vi "Dashboard Main.vi"() -> ()   [LabVIEW 2017]
uses:
  <vilib>/Utility/miscctls.llb/LVRowAndColumnTypeDef.ctl
  <vilib>/event_ctls.llb/eventvkey.ctl
  <vilib>/Rock Robotics/Network Tables/NT Read Numeric Array.vi
  <vilib>/Rock Robotics/WPI/Dashboard/WPI_DashboardLogging Global.vi
panel:
  in  "Camera Settings Right":T1={"Frame Rate"=30, "Compression"=30, "Size"=1, "DB Camera Config"=FALSE} {"Frame Rate" scale=1.0..30.0; "Compression" scale=100.0..-1.0; "Size" items=["640x480", "320x240", "160x120"]}
  in  "Camera Name Right":string(combo)="No Camera Selection"
  out "Camera Info":cluster{"Mbps LED":bool, "Mbps":dbl, "fps":dbl} {"fps" format="%#.1g"; "Mbps" format="%#.1g"}
  in  "Camera Settings":T1={"Frame Rate"=30, "Compression"=30, "Size"=1, "DB Camera Config"=FALSE} {"Frame Rate" scale=1.0..30.0; "Compression" scale=100.0..-1.0; "Size" items=["640x480", "320x240", "160x120"]}
  in  "TCP":refnum<k5>
  in  "Rec Mode":enum32{"Stop", "Record", "Playback"}(radio)
  out "Robot IP":string
  out "Image Message":string="Timeout in Camera Communications"
  in  "Dashboard Tab":T2(tab)=enum."Custom"
  in  "Select Auto":string(combo)="Select Autonomous ..."
  out "NT Connection":bool
  out "MotorChart R":cluster{"Numeric":dbl, "Numeric":dbl}(graph)
  out "MotorChart L":cluster{"Numeric":dbl, "Numeric":dbl}(graph)
  out "MotorSliders R":cluster{"MotorSlide1":dbl, "MotorSlide2":dbl} {"MotorSlide2" scale=-1.0..1.0 scale format="%#_2e"; "MotorSlide1" scale=-1.0..1.0 scale format="%#_2e"}
  out "MotorSliders L":cluster{"MotorSlide1":dbl, "MotorSlide2":dbl} {"MotorSlide2" scale=-1.0..1.0 scale format="%#_2e"; "MotorSlide1" scale=-1.0..1.0 scale format="%#_2e"}
  out "Gyro":dbl(knob) scale=0.0..360.0
  out "JS1 Z":dbl(slide) scale=-1.0..1.0 scale format="%#_2e"
  out "JS1 Graph":cluster{"X":dbl, "Y":dbl}[](graph)
  out "JS1 Buttons":T3
  out "JS2 Z":dbl(slide) scale=-1.0..1.0 scale format="%#_2e"
  out "JS2 Graph":cluster{"X":dbl, "Y":dbl}[](graph)
  out "JS2 Buttons":T3
  out "Mode":T4(ring)=enum."Auto Disabled"
  out "Camera Image Right":T5(plugin-control)
  in  "DB/String 9":string
  in  "DB/String 8":string
  in  "DB/String 7":string
  in  "DB/String 6":string
  in  "DB/String 5":string
  in  "DB/String 4":string
  in  "DB/String 3":string
  in  "DB/String 2":string
  in  "DB/String 1":string
  in  "DB/String 0":string
  in  "DB/Slider 0":dbl(slide) scale=0.0..5.0
  in  "DB/Slider 1":dbl(slide) scale=0.0..5.0
  in  "DB/Slider 2":dbl(slide) scale=0.0..5.0
  in  "DB/Slider 3":dbl(slide) scale=0.0..5.0
  out "DB/LED 3":bool
  out "DB/LED 2":bool
  out "DB/LED 1":bool
  out "DB/LED 0":bool
  in  "DB/Button 3":bool
  in  "DB/Button 2":bool
  in  "DB/Button 1":bool
  in  "DB/Button 0":bool caption="New Name"
  in  "Turning Deadband":dbl
  in  "Turning Rate":dbl
  in  "Speed Deadband":dbl
  in  "Speed Rate":dbl
  in  "Climb Time":dbl
  in  "Climb Setpoint":dbl=0.7
  in  "Button Lower Arm Time":dbl
  in  "Button Lower Arm Setpoint":dbl=0.7
  in  "Button Lift Arm Time":dbl
  in  "Button Lift Arm Setpoint":dbl=0.7
  in  "Release Time":dbl
  in  "Release Setpoint":dbl=0.7
  in  "Grab Setpoint":dbl=0.7
  in  "Grab Time":dbl=1.0
  in  "Test Slider":dbl(slide) scale=0.0..100.0 scale format="%#_3g"
  in  "On/Off":bool caption="Solenoid"
  in  "Test Name":u16(ring) items=["Select the test to run..."]
  in  "Test Tree":string(tree)
  in  "Motor":cluster{"Value":dbl, "Enable":bool} {"Value" scale=-1.0..1.0 scale format="%#_3g"}
  out "Progress":T6 {"Test Progress" scale=0.0..100.0}
  in  "Rev/Fwd":cluster{"Forward":bool, "Reverse":bool}
  in  "Test Ring":u16(ring) items=["Monochrome", "Color"]
  out "Cmd Status":string
  in  "Execute Command":bool
  in  "Command Params":string[][](table)
  in  "Command Selection":i32(listbox)
  in  "CheckList":i32(listbox)
  out "Tree":string(tree)
  out "Camera Image":T5(plugin-control)
  out "Background":bool
  in  "Camera Name":string(combo)="No Camera Selection"
  # "HW"
  # "HW"
  # "Joysticks"
  # "Drive Motors"
  # "Front"
  # "Right"
  # "Left"
  # "Back"
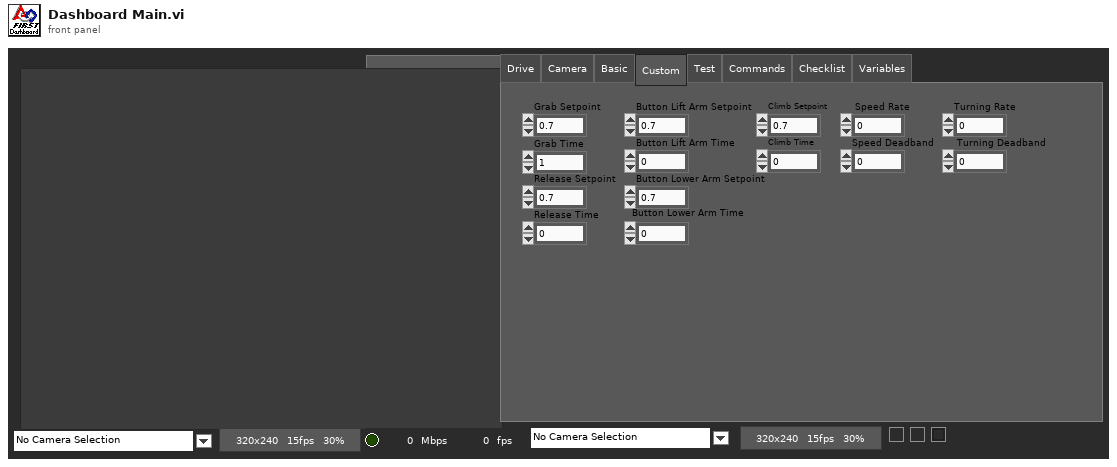
[diagram p1: front panel]
types:
  T1 = cluster{"Frame Rate":i32, "Compression":i32, "Size":u16, "DB Camera Config":bool}
  T2 = enum32{"Drive", "Camera", "Basic", "Custom", "Test", "Commands", "Checklist", "Variables"}
  T3 = cluster{bool, bool, bool, bool, bool, bool, bool, bool, bool, bool, bool, bool}
  T4 = enum8{"Tele-Op Disabled", "Tele-Op Enabled", "Auto Disabled", "Auto Enabled", "Test Disabled", "Test Enabled", "Disconnected", "No Code", "E-Stop"}
  T5 = typedef "IMAQ Image.ctl" = refnum<image>
  T6 = cluster{"Test Progress":u8, "Test Progress Text":string}
  T7 = cluster{"Save Path":path, "Interval (s)":dbl, "Keep":i32}
  T8 = typedef "Image Type" = u32
  T9 = cluster{"IDs":cluster{"RPC field ID":u16, "Unique ID":u16}, "String":string}
  T10 = cluster{"Error Strings":string, "Disable Counts":cluster{u16, u16}, "Rail Faults":cluster{u16, u16, u16}, "Robot IP":string, "DB Mode":u8, "Event Info":cluster{"Name":string, "Type":u8, "Number":u16, "Replay":u8}}
  T11 = cluster{"Storage":cluster{"Disk Free":u64, "RAM Block":u32, "RAM free":u32}, "CPU Utilization":cluster{"CPU % ISR":sgl, "CPU % Time Crit":sgl, "CPU % Timed Str":sgl, "CPU % High":sgl, "CPU % Above":sgl, "CPU % Normal":sgl, "CPU % Low":sgl}, "CAN":cluster{"% Bus Utilization":sgl, "Bus Off Cnt":u32, "TX_FIFO Full Cnt":u32, "Receive Error Cnt":u8, "Transmit Error Cnt":u8}, "HID":cluster{"HID Outputs":u32, "Rumble Low":u16, "Rumble High":u16}[]}
  T12 = cluster{"Status bits":cluster{"Test Mode":bool, "Autonomous":bool, "Enabled":bool, "Code Start":bool, "Brownout":bool, "Reserved 2":bool, "Reserved 3":bool, "E-Stop":bool}, "Code Trace":cluster{"Disabled":bool, "TeleOp":bool, "Auto":bool, "Test":bool}, "Controller Type":enum16{"unknown", "cRIO", "roboRio"}, "Code?":enum16{"unknown", "noCode", "code"}, "Battery V":dbl}
  T13 = cluster{"Control Bits":cluster{"TestMode":bool, "Autonomous":bool, "Enabled":bool, "FMS Present":bool, bool, bool, bool, "E-Stop":bool}, "Team Station ":u8, "Countdown":sgl, "Joystick Values":cluster{"Axes":dbl[], "Buttons":bool[], "POVs":i16[]}[]}
  T14 = cluster{"Axes":dbl[], "Buttons":bool[], "POVs":i16[]}[]
  T15 = cluster{"Axes":dbl[], "Buttons":bool[], "POVs":i16[]}
  T16 = cluster{"Buttons[0]":bool, "Buttons[1]":bool, "Buttons[2]":bool, "Buttons[3]":bool, "Buttons[4]":bool, "Buttons[5]":bool, "Buttons[6]":bool, "Buttons[7]":bool, "Buttons[8]":bool, "Buttons[9]":bool, "Buttons[10]":bool, "Buttons[11]":bool}
  T17 = cluster{"Camera Image":refnum<vi>, "Dashboard Tab":refnum<vi>, "Background":refnum<vi>, "Rec Mode":refnum<vi>, "Test Slider":refnum<vi>, "On/Off ":refnum<vi>, "Test Ring":refnum<vi>, "Rev/Fwd":refnum<vi>, "Test Name":refnum<vi>, "Motor":refnum<vi>, "Progress":refnum<vi>, "CheckList":refnum<vi>, "Tree":refnum<vi>, "Test Tree":refnum<vi>, "Command Params":refnum<vi>, "Command Selection":refnum<vi>, "Execute Command":refnum<vi>, "Cmd Status":refnum<vi>, "Camera Settings":refnum<vi>, "Camera Name":refnum<vi>, "Camera Info":refnum<vi>, "Camera Settings Right":refnum<vi>, "Camera Name Right":refnum<vi>, "Camera Image Right":refnum<vi>}
  T18 = cluster{"Camera Name":string, string, "Saved DB Images Info":cluster{"Save Path":path, "Interval (s)":dbl, "Keep":i32}}
  T19 = cluster{"Camera Name Right":string, string, "Saved DB Images Info":cluster{"Save Path":path, "Interval (s)":dbl, "Keep":i32}}
  T20 = cluster{"Operation":enum16{"Update", "Clear"}, "Color Box":u32}[]
  T21 = typedef "eventvkey.ctl" = enum16{"ASCII", "Enter", "Return", "Shift", "Ctrl", "Alt", "Cmd", "Opt", "Caps", "NumLock", "Clear", "Break", "Up", "Down", "Left", "Right", "Insert", "Delete", "Home", "End", "PageUp", "PageDown", "Escape", "Help", "Pause", "ScrollLock", "F1", "F2", "F3", "F4", "F5", "F6", "F7", "F8", "F9", "F10", "F11", "F12", "F13", "F14", "F15", "F16", "F17", "F18", "F19", "F20", "F21", "F22", "F23", "F24", "Play", "VolumeUp", "VolumeDown", "Mute", "Two Byte Char"}
  T22 = cluster{"Image Size":bool, "Image Type":bool, "Pixel Value":bool, "ROI Information":bool, "Zoom Factor":bool}
  T23 = cluster{"Operation":enum16{"Update", "Clear"}, "Color Box":u32}
  T24 = typedef "LVRowAndColumnTypeDef.ctl" = cluster{"Row":i32, "Column":i32}
  T25 = cluster{"Shift":bool, "Ctrl":bool, "Alt":bool, "Cmd":bool, "Opt":bool}
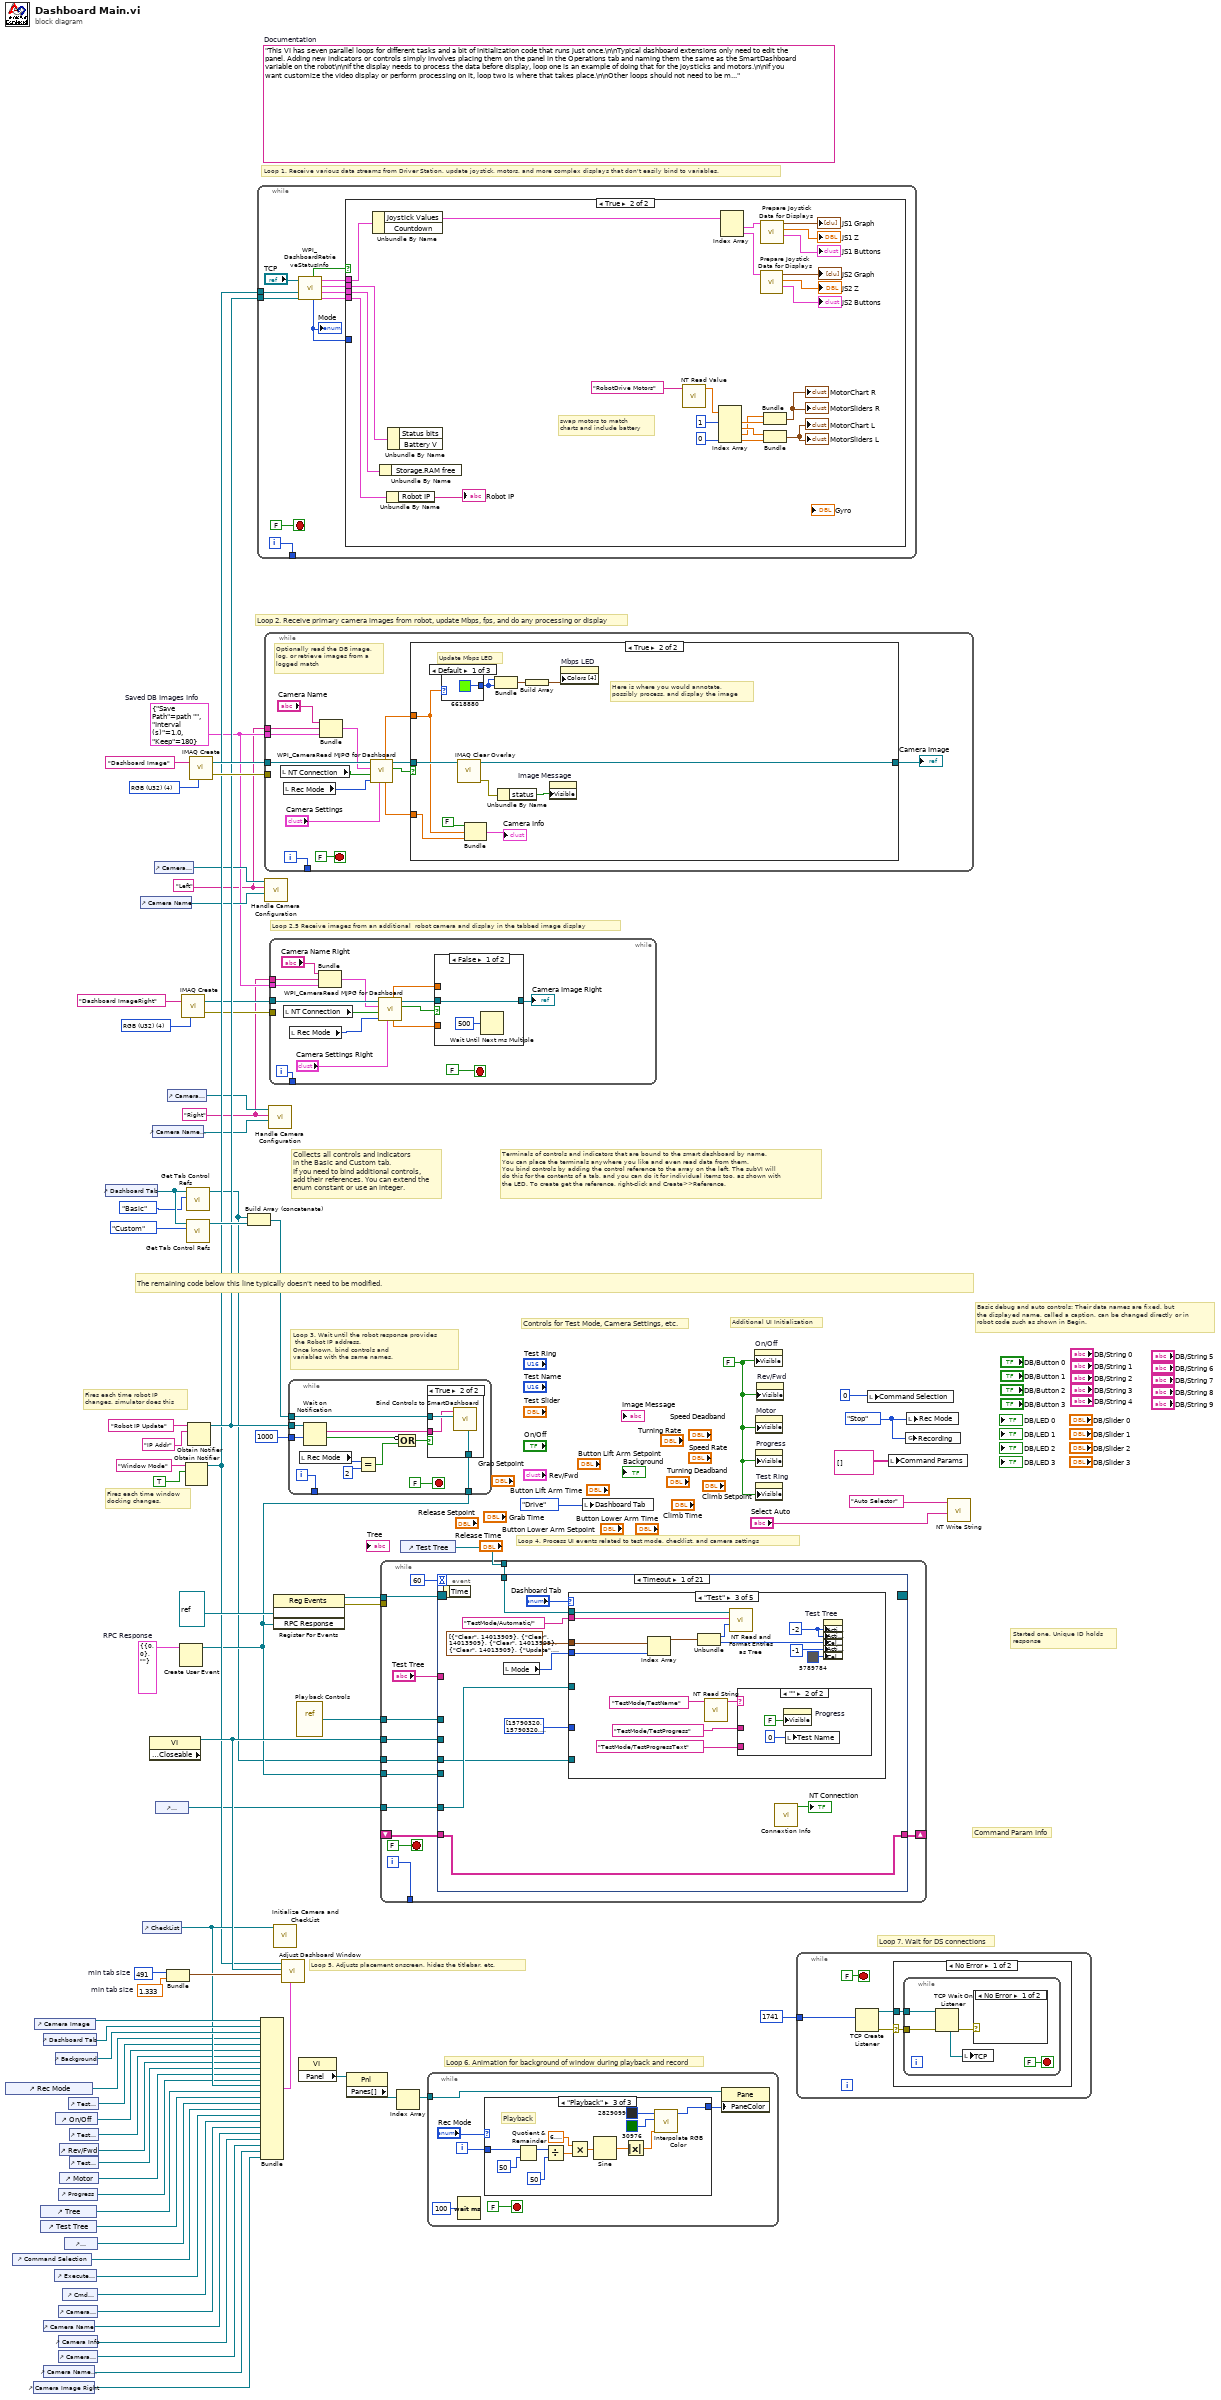
[diagram p0: block diagram]
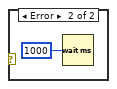
[diagram p3: hidden frame]
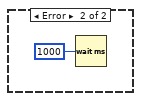
[diagram p4: hidden frame]
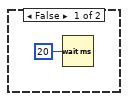
[diagram p5: hidden frame]
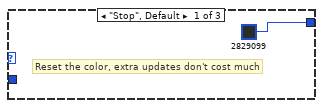
[diagram p6: hidden frame]
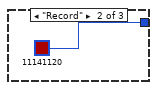
[diagram p7: hidden frame]
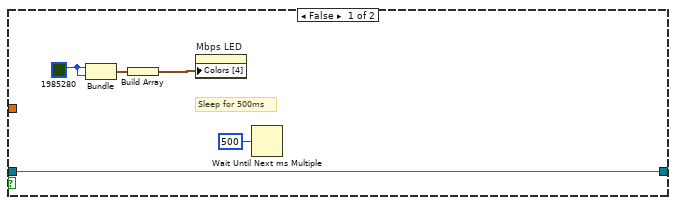
[diagram p9: hidden frame]
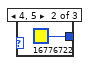
[diagram p10: hidden frame]
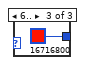
[diagram p11: hidden frame]
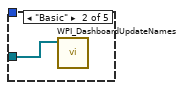
[diagram p13: hidden frame]
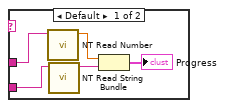
[diagram p14: hidden frame]
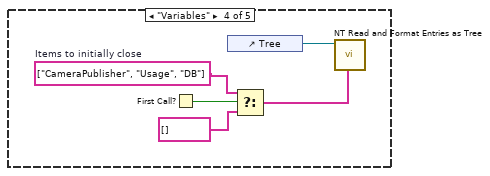
[diagram p15: hidden frame]
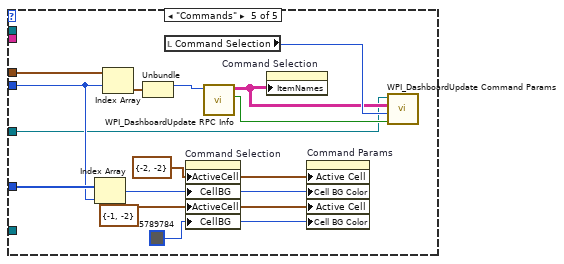
[diagram p16: hidden frame]
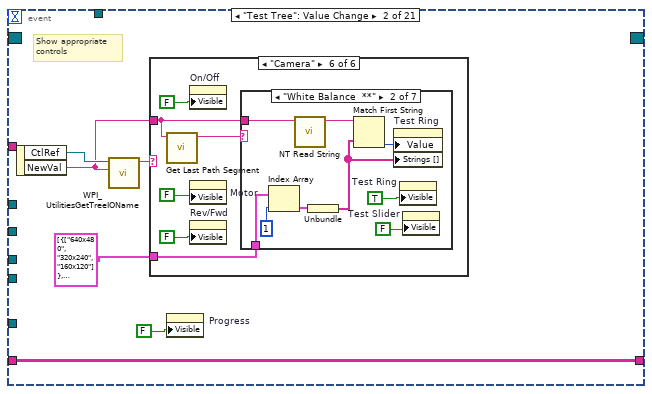
[diagram p17: hidden frame]
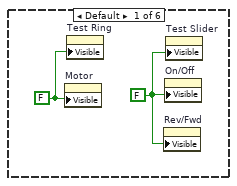
[diagram p18: hidden frame]
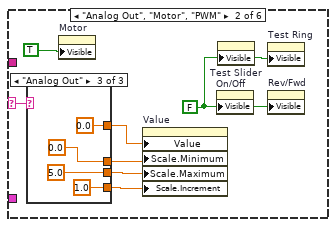
[diagram p19: hidden frame]
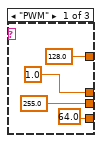
[diagram p20: hidden frame]
diagram:
  w3 = T7 {"Save Path"=path "", "Interval (s)"=1.0, "Keep"=180}  # Saved DB Images Info
  w2 = "Right"
  w1 = "Left"
  w13 = T8 4 items=["Grayscale (U8)", "Grayscale (I16)", "Grayscale (SGL)", "Complex (CSG)", "RGB (U32)", "HSL (U32)", "RGB (U64)"] ("Image Type")
  w29 = T9 {"IDs"={"RPC field ID"=0, "Unique ID"=0}, "String"=""}  # RPC Response
  w52 = 491  # min tab size
  w51 = 1.333  # min tab size
  w59 = enum32{"Stop", "Record", "Playback"}."Stop" ("Rec Mode")
  w36 = FALSE ("Visible")
  (unwired) "This VI has seven parallel loops for different tasks and a bit of initialization code that runs just once.\n\nTypical dashboard extensions only need to edit the panel. Adding new indicators or controls simply involves placing them on the panel in the Operations tab and naming them the same as the SmartDashboard variable on the robot\n\nIf the display needs to process the data before display, loop one is an example of doing that for the joysticks and motors.\n\nIf you want customize the video display or perform processing on it, loop two is where that takes place.\n\nOther loops should not need to be modified. They are pretty standard, and document the task they perform."  # Documentation
  w76 = T8 4 items=["Grayscale (U8)", "Grayscale (I16)", "Grayscale (SGL)", "Complex (CSG)", "RGB (U32)", "HSL (U32)", "RGB (U64)"] ("Image Type")
  # "Loop 2.5 Receive images from an additional  robot camera and display in the tabbed image display"
  # "Command Param Info"
  # "Started one, Unique ID holds\nresponse"
  # "Loop 7. Wait for DS connections"
  # "Basic debug and auto controls: Their data names are fixed, but\nthe displayed name, called a caption, can be changed directly or in\nrobot code such as shown in Begin."
  # "Controls for Test Mode, Camera Settings, etc."
  # "Additional UI Initialization"
  # "Loop 6. Animation for background of window during playback and record"
  # "Fires each time robot IP\nchanges, simulator does this"
  # "Fires each time window\ndocking changes."
  # "Collects all controls and indicators\nin the Basic and Custom tab.\nIf you need to bind additional controls,\nadd their references. You can extend the\nenum constant or use an integer."
  # "The remaining code below this line typically doesn't need to be modified."
  # "Loop 4. Process UI events related to test mode, checklist, and camera settings"
  # "Terminals of controls and indicators that are bound to the smart dashboard by name.\nYou can place the terminals anywhere you like and even read data from them.\nYou bind controls by adding the control reference to the array on the left. The subVI will\ndo this for the contents of a tab, and you can do it for individual items too, as shown with\nthe LED. To create get the reference, right-click and Create>>Reference."
  # "Loop 3. Wait until the robot response provides\n the Robot IP address.\nOnce known, bind controls and\nvariables with the same names."
  # "Loop 5. Adjusts placement onscreen, hides the titlebar, etc."
  # "Loop 1. Receive various data streams from Driver Station, update joystick, motors, and more complex displays that don't easily bind to variables."
  # "Loop 2. Receive primary camera images from robot, update Mbps, fps, and do any processing or display"
  n1 = control-ref of="Rec Mode"() -> (w42:refnum<vi>)
  n2 = control-ref of="Command Selection"() -> (w28:refnum<vi>)
  n3 = control-ref of="Camera Image Right"() -> (w6:refnum<vi>)
  n4 = control-ref of="Camera Image"() -> (w54:refnum<vi>)
  n5 = control-ref of="Tree"() -> (w46:refnum<vi>)
  n6 = control-ref of="Test Tree"() -> (w45:refnum<vi>)
  n7 = control-ref of="Dashboard Tab"() -> (w53:refnum<vi>)
  n8 = control-ref of="Camera Name"() -> (w19:refnum<vi>)
  n9 = control-ref of="Camera Name Right"() -> (w7:refnum<vi>)
  n10 = control-ref of="Execute Command"() -> (w30:refnum<vi>)
  n11 = control-ref of="Background"() -> (w49:refnum<vi>)
  n12 = control-ref of="On/Off"() -> (w40:refnum<vi>)
  n13 = control-ref of="Progress"() -> (w37:refnum<vi>)
  n14 = control-ref of="Camera Settings"() -> (w20:refnum<vi>)
  n15 = control-ref of="Camera Info"() -> (w18:refnum<vi>)
  n16 = control-ref of="Camera Settings Right"() -> (w8:refnum<vi>)
  n17 = control-ref of="Rev/Fwd"() -> (w38:refnum<vi>)
  n18 = control-ref of="Motor"() -> (w43:refnum<vi>)
  n19 = control-ref of="Cmd Status"() -> (w24:refnum<vi>)
  n20 = control-ref of="Command Params"() -> (w31:refnum<vi>)
  n21 = control-ref of="Test Slider"() -> (w41:refnum<vi>)
  n22 = control-ref of="Test Ring"() -> (w39:refnum<vi>)
  n23 = control-ref of="Test Name"() -> (w44:refnum<vi>)
  n24 = control-ref of="Dashboard Tab"() -> (w57:refnum<vi>)
  n25 = control-ref of="Camera Name"() -> (w21:refnum<vi>)
  n26 = control-ref of="CheckList"() -> (w47:refnum<vi>)
  n27 = property class="VI" props=["Front Panel.Closeable"]() -> (reference out=w58:refnum<vi>)  [unwired: 2 in, 2 out]
  n28 = control-ref of="Camera Name Right"() -> (w9:refnum<vi>)
  n29 = control-ref of="Camera Settings"() -> (w22:refnum<vi>)
  n30 = control-ref of="Command Params"() -> (w23:refnum<vi>)
  n31 = Bundle("min tab size"=w52, "min tab size"=w51) -> (w50:cluster{"min tab size":i32, "min tab size":dbl})  [unwired: 1 in]
  n32 = control-ref of="Camera Settings Right"() -> (w10:refnum<vi>)
  n33 = Create User Event(user event datatype=w29) -> (user event=w25:refnum<user-event>)  [unwired: 1 in, 1 out]
  n34 = call "IMAQ Create"("Image Name"="Dashboard ImageRight", "Image Type"=w13) -> ("New Image"=w12:T5, "error out"=w11:errorcluster)  [unwired: 2 in, 1 out]
  n35 = Obtain Notifier(name (unnamed)="Window Mode", notification data type=TRUE) -> (notifier out=w34:refnum<notifier>)  [unwired: 2 in, 2 out]
  n36 = call <vilib>:"Get Tab Control Refs.vi"("Page Index"=T2."Basic" ("Dashboard Tab"), "TabControl in"=w57) -> ("ControlsOnPage"=w17:refnum<vi>[])  [unwired: 9 in]
  n37 = call <vilib>:"Get Tab Control Refs.vi"("Page Index"=T2."Custom" ("Dashboard Tab"), "TabControl in"=w57) -> ("ControlsOnPage"=w56:refnum<vi>[])  [unwired: 9 in]
  n38 = Obtain Notifier(name (unnamed)="Robot IP Update", notification data type="IP Addr" ("name (unnamed)")) -> (notifier out=w35:refnum<notifier>)  [unwired: 2 in, 2 out]
  n39 = call "IMAQ Create"("Image Name"="Dashboard Image", "Image Type"=w76) -> ("New Image"=w74:T5, "error out"=w73:errorcluster)  [unwired: 2 in, 1 out]
  n40 = Build Array (concatenate)(w17, w56) -> (w55:refnum<vi>[])
  n41 = while {
    tunnel: [w86] -> _
    tunnel: w35 -> [w80]
    tunnel: w34 -> [w77]
    i -> [w86]
    stop <- FALSE stop-if-true
    n42 = call <vilib>:"WPI_DashboardRetrieveStatusInfo.vi"("Binding Refnum"=w80, "Window Mode Notifier"=w77, "TCP Cnx"="TCP") -> ("Power and Errors"=w81:T10, "Robot Metrics"=w84:T11, "Status Info"=w85:T12, "Control Info"=w82:T13, "Robot Mode"=w79:T4, "Process?"=w83:bool)  [unwired: 3 in]
    "Mode" <- w79
    n43 = case shown="True" w83 {
      tunnel: w85 -> [_ w112]
      tunnel: w84 -> [_ w111]
      tunnel: w82 -> [_ w110]
      tunnel: w81 -> [_ w109]
      tunnel: w79 -> [_ _]
      frame False {
        n44 = Wait (ms)(milliseconds to wait=u32 20) -> ()  [unwired: 1 out]
      }
      frame True {
        # "swap motors to match\ncharts and include battery"
        n45 = Unbundle By Name(w110) -> ("Joystick Values"=w100:T14)  [unwired: 1 out]
        n46 = Unbundle By Name(w111) -> ()  [unwired: 1 out]
        n47 = Unbundle By Name(w109) -> ("Robot IP"=→"Robot IP":string)
        n48 = Unbundle By Name(w112) -> ()  [unwired: 2 out]
        n49 = call-poly <vilib>:"NT Read Value.vi"("Name"="RobotDrive Motors") -> ("Numeric Array"=w90:dbl[])  [unwired: 9 in, 1 out]
        n50 = Index Array(array=w90, index #1=1, index #4=0) -> (element #1=w104:dbl, element #2=w105:dbl, element #3=w103:dbl, element #4=w108:dbl)  [unwired: 2 in]
        n51 = Index Array(array=w100) -> (element #1=w99:T15, element #2=w95:T15)  [unwired: 2 in]
        n52 = call "Prepare Joystick Data for Displays.vi"("Joystick Values"=w95) -> ("Buttons"=→"JS2 Buttons":T16, "Z Axis"=→"JS2 Z":dbl, "Cartesian Data"=→"JS2 Graph":cluster{"X axis":dbl, "X axis":dbl}[])  [unwired: 8 in]
        n53 = call "Prepare Joystick Data for Displays.vi"("Joystick Values"=w99) -> ("Buttons"=→"JS1 Buttons":T16, "Z Axis"=→"JS1 Z":dbl, "Cartesian Data"=→"JS1 Graph":cluster{"X axis":dbl, "X axis":dbl}[])  [unwired: 8 in]
        n54 = Bundle("Numeric"=w103, "Numeric"=w104) -> (→"MotorChart R" →"MotorSliders R":cluster{"Numeric":dbl, "Numeric":dbl})  [unwired: 1 in]
        n55 = Bundle("Numeric"=w105, "Numeric"=w108) -> (→"MotorChart L" →"MotorSliders L":cluster{"Numeric":dbl, "Numeric":dbl})  [unwired: 1 in]
      }
    }
  }
  n56 = Bundle("Camera Image"=w54, "Dashboard Tab"=w53, "Background"=w49, "Rec Mode"=w42, "Test Slider"=w41, "On/Off"=w40, "Test Ring"=w39, "Rev/Fwd"=w38, "Test Name"=w44, "Motor"=w43, "Progress"=w37, "CheckList"=w47, "Tree"=w46, "Test Tree"=w45, "Command Params"=w31, "Command Selection"=w28, "Execute Command"=w30, "Cmd Status"=w24, "Camera Settings"=w20, "Camera Name"=w19, "Camera Info"=w18, "Camera Settings Right"=w8, "Camera Name Right"=w7, "Camera Image Right"=w6) -> (w48:T17)  [unwired: 1 in]
  n57 = call "Handle Camera Configuration.vi"("CameraNameRef"=w21, "Display Name"=w1, "ClusterRef"=w22) -> ()  [unwired: 9 in]
  n58 = while {
    tunnel: w74 -> [w125]
    tunnel: w73 -> [_]
    tunnel: [w126] -> _
    tunnel: w3 -> [w116]
    tunnel: w1 -> [w113]
    i -> [w126]
    stop <- FALSE stop-if-true
    # "Optionally read the DB image,\nlog, or retrieve images from a\nlogged match"
    n59 = local read "NT Connection"() -> (w117:bool)
    n60 = local read "Rec Mode"() -> (w121:enum32{"Stop", "Record", "Playback"})
    n61 = Bundle("Camera Name"="Camera Name", w113, "Saved DB Images Info"=w116) -> (w115:T18)  [unwired: 1 in]
    n62 = call <vilib>:"WPI_CameraRead MJPG for Dashboard.vi"("Camera Settings"="Camera Settings", "Rec Mode"=w121, "NT Connection"=w117, "Capture Info"=w115, "Refnum in"=w125) -> ("Active"=w123:bool, "Refnum out"=w124:T5, "FPS"=w122:dbl, "Bandwidth (Mbps)"=w120:dbl)  [unwired: 3 in]
    n63 = case shown="True" w123 {
      tunnel: w124 -> [w128 w139]
      tunnel: w120 -> [_ w136]
      tunnel: w122 -> [_ w137]
      tunnel: [w128 w133] -> w118
      frame False {
        w130 = u32 1985280 ("Color Box")
        # "Sleep for 500ms"
        n64 = Bundle("Color Box"=w130, "Color Box"=w130) -> (w131:cluster{"Color Box":u32, "Color Box":u32})  [unwired: 1 out]
        n65 = Build Array(w131) -> (w129:cluster{"Color Box":u32, "Color Box":u32}[])
        n66 = property on="Mbps LED" class="Bool (strict)"("Colors [4]"=w129) -> ()  [unwired: 2 in, 2 out]
        n67 = Wait Until Next ms Multiple(millisecond multiple=u32 500) -> ()  [unwired: 1 out]
      }
      frame True {
        # "Here is where you would annotate,\npossibly process, and display the image"
        # "Update Mbps LED"
        n68 = case shown="Default" w136 {
          tunnel: [u32 6618880 ("Color Box") u32 16776722 ("Color Box") u32 16716800 ("Color Box")] -> w140
          frame Default {
          }
          frame 4, 5 {
          }
          frame 6.. {
          }
        }
        n69 = call "IMAQ Clear Overlay"("Image"=w139) -> ("error out"=w142:errorcluster, "Image Out"=w133:T5)  [unwired: 2 in, 7 out]
        n70 = Bundle(FALSE, "Bandwidth (Mbps)"=w136, "FPS"=w137) -> (→"Camera Info":cluster{bool, "Bandwidth (Mbps)":dbl, "FPS":dbl})  [unwired: 1 in]
        n71 = Bundle("Color Box"=w140, "Color Box"=w140) -> (w141:cluster{"Color Box":u32, "Color Box":u32})  [unwired: 1 out]
        n72 = Unbundle By Name(w142) -> ("status"=w143:bool)
        n73 = Build Array(w141) -> (w138:cluster{"Color Box":u32, "Color Box":u32}[])
        n74 = property on="Image Message" class="Str"("Visible"=w143) -> ()  [unwired: 2 in, 2 out]
        n75 = property on="Mbps LED" class="Bool (strict)"("Colors [4]"=w138) -> ()  [unwired: 2 in, 2 out]
      }
    }
    "Camera Image" <- w118
  }
  n76 = call "Handle Camera Configuration.vi"("CameraNameRef"=w9, "Display Name"=w2, "ClusterRef"=w10) -> ()  [unwired: 9 in]
  n77 = while {
    tunnel: w12 -> [w161]
    tunnel: w11 -> [_]
    tunnel: [w156] -> _
    tunnel: w3 -> [w150]
    tunnel: w2 -> [w147]
    i -> [w156]
    stop <- FALSE stop-if-true
    n78 = local read "NT Connection"() -> (w151:bool)
    n79 = local read "Rec Mode"() -> (w160:enum32{"Stop", "Record", "Playback"})
    n80 = Bundle("Camera Name Right"="Camera Name Right", w147, "Saved DB Images Info"=w150) -> (w149:T19)  [unwired: 1 in]
    n81 = call <vilib>:"WPI_CameraRead MJPG for Dashboard.vi"("Camera Settings"="Camera Settings Right", "Rec Mode"=w160, "NT Connection"=w151, "Capture Info"=w149, "Refnum in"=w161) -> ("Active"=w155:bool, "Refnum out"=w158:T5, "FPS"=w153:dbl, "Bandwidth (Mbps)"=w154:dbl)  [unwired: 3 in]
    n82 = case shown="False" w155 {
      tunnel: w158 -> [w162 w164]
      tunnel: w154 -> [_ _]
      tunnel: w153 -> [_ _]
      tunnel: [w162 w164] -> w152
      frame False {
        n83 = Wait Until Next ms Multiple(millisecond multiple=u32 500) -> ()  [unwired: 1 out]
      }
      frame True {
      }
    }
    "Camera Image Right" <- w152
  }
  n84 = register-events(refnum<vi> refnum, w25) -> (reference out=w63:refnum<event-registration>, error out=w62:errorcluster)  [unwired: 2 in]
  n85 = call "Initialize Camera and CheckList.vi"("ListBox in"=w47) -> ()  [unwired: 11 in]
  n86 = call "Adjust Dashboard Window.vi"("Sizing Refnums"=w48, "Size Constraints"=w50, "VI"=w58, "WIn Mode"=w34) -> ()  [unwired: 8 in]
  n87 = while {
    tunnel: w55 -> [w176]
    tunnel: w35 -> [w174]
    tunnel: [w172] -> _
    tunnel: u32 1000 ("milliseconds to wait") -> [w171]
    tunnel: w25 -> [w165]
    i -> [w172]
    stop <- FALSE stop-if-true
    n88 = local read "Rec Mode"() -> (w167:enum32{"Stop", "Record", "Playback"})
    n89 = Wait on Notification(notifier=w174, timeout in ms (-1)=w171) -> (notification=w173:string, timed out?=w169:bool)  [unwired: 2 in, 2 out]
    n90 = Equal?(x=w167, y=u16 2 ("Rec Mode")) -> (x = y?=w168:bool)
    n91 = Compound Arithmetic op=OR(invert w169, w168) -> (w170:bool)
    n92 = case shown="True" w170 {
      tunnel: w176 -> [_ w179]
      tunnel: w173 -> [_ w178]
      tunnel: w165 -> [_ w177]
      frame False {
      }
      frame True {
        n93 = call <vilib>:"Bind Controls to SmartDashboard.vi"("RPC ref"=w177, "Bound Control Refs"=w179, "Server IP Address"=w178) -> ()  [unwired: 9 in]
      }
    }
  }
  n94 = vi-ref "Playback Controls.vi"() -> (w64:refnum<vi>)
  n95 = property class="VI"() -> ("Panel"=w66:refnum<vi>)  [unwired: 2 in, 2 out]
  n96 = property class="Pnl"(reference=w66) -> ("Panes[]"=w67:refnum<vi>[])  [unwired: 1 in, 2 out]
  n97 = Index Array(array=w67) -> (element=w65:refnum<vi>)  [unwired: 1 in]
  n98 = control-ref of="Test Tree"() -> (w68:refnum<vi>)
  n99 = while {
    tunnel: [w189] -> _
    tunnel: w68 -> [w188]
    tunnel: w64 -> [w187]
    tunnel: w63 -> [w186]
    tunnel: w62 -> [_]
    tunnel: w58 -> [w185]
    tunnel: w25 -> [w184]
    tunnel: w23 -> [w183]
    shift-right: [w182] -> _
    shift-left: _ -> [w181]
    tunnel: w17 -> [w180]
    i -> [w189]
    stop <- FALSE stop-if-true
    n100 = event shown="[0] Timeout" {
      selector: w186 -> [_ _ _ _ _ _ _ _ _ _ _ _ _ _ _ _ _ _ _ _ _]
      dyn-events: [_ _ _ _ _ _ _ _ _ _ _ _ _ _ _ _ w449 _ _ _ _] -> _
      timeout: u32 60 ("milliseconds to wait") -> [_ _ _ _ _ _ _ _ _ _ _ _ _ _ _ _ _ _ _ _ _]
      tunnel: w188 -> [w201 _ _ _ _ _ _ _ _ _ _ _ _ _ _ _ _ _ _ _ _]
      tunnel: "Test Tree" -> [_ _ _ _ _ _ _ _ _ _ _ w416 w424 w426 w430 w438 _ _ _ _ _]
      tunnel: w187 -> [_ _ _ _ _ _ _ _ _ _ _ _ _ _ _ _ w451 _ w469 _ _]
      tunnel: w185 -> [_ _ _ _ _ _ _ _ _ _ _ _ _ _ _ _ w447 _ _ _ _]
      tunnel: w184 -> [_ _ _ _ _ _ _ _ _ _ _ _ _ _ _ _ w445 _ _ _ _]
      tunnel: w183 -> [w196 _ _ _ _ _ w367 _ _ _ _ _ _ _ _ _ _ _ _ _ _]
      tunnel: [w195 w244 w346 w351 w360 w364 w365 w374 w384 w391 w403 w415 w422 w425 w429 w437 w444 w464 w466 w470 w483] -> w182
      tunnel: w181 -> [w195 w244 w346 w351 w360 w364 w365 _ _ w391 w403 w415 w422 w425 w429 w437 w444 w464 w466 w470 w483]
      tunnel: w180 -> [w193 _ _ _ _ _ _ _ _ _ _ _ _ _ _ _ _ _ _ _ _]
      event Timeout {
        n101 = event-data() -> ()  [unwired: 1 in, 1 out]
        n102 = local read "Mode"() -> (w198:T4)
        n103 = case shown="\"Test\"" "Dashboard Tab" {
          tunnel: w201 -> [_ _ w217 _ _]
          tunnel: "TestMode/Automatic/" ("Name Pattern") -> [_ _ w216 _ _]
          tunnel: T20 [{"Operation"=enum."Clear", "Color Box"=14013909}, {"Operation"=enum."Clear", "Color Box"=14013909}, {"Operation"=enum."Clear", "Color Box"=14013909}, {"Operation"=enum."Clear", "Color Box"=14013909}, {"Operation"=enum."Update", "Color Box"=14013909}, {"Operation"=enum."Update", "Color Box"=16777215}, {"Operation"=enum."Clear", "Color Box"=14013909}, {"Operation"=enum."Clear", "Color Box"=14013909}, {"Operation"=enum."Clear", "Color Box"=14013909}] -> [_ _ w209 _ w237]
          tunnel: w198 -> [_ _ w208 _ w236]
          tunnel: u32[] [15790320, 15790320, 15790320, 15790320, 16777215, 16777215, 15790320, 15790320, 15790320] -> [_ _ _ _ w242]
          tunnel: w196 -> [_ _ _ _ w230]
          tunnel: w193 -> [_ w203 _ _ _]
          frame "Custom", Default {
          }
          frame "Basic" {
            n104 = call <vilib>:"WPI_DashboardUpdateNames.vi"("Controls on Tab"=w203) -> ()  [unwired: 11 in]
          }
          frame "Test" {
            w215 = -2 ("Active Item:Row Number")
            n105 = Index Array(array=w209, index=w208) -> (element=w210:T23)
            n106 = Unbundle(w210) -> ("Operation"=w211:enum16{"Update", "Clear"}, "Color Box"=w212:u32)
            n107 = call <vilib>:"NT Read String.vi"("Name"="TestMode/TestName") -> ("String"=w206:string)  [unwired: 9 in, 1 out]
            n108 = call <vilib>:"NT Read and Format Entries as Tree.vi"("Operation"=w211, "Name Pattern"=w216, "Tree Refnum"=w217) -> ()  [unwired: 7 in, 2 out]
            n109 = case shown="\"\"" w206 {
              tunnel: "TestMode/TestProgress" ("Name") -> [w219 _]
              tunnel: "TestMode/TestProgressText" ("Name") -> [w218 _]
              frame Default {
                n110 = call <vilib>:"NT Read Number.vi"("Name"=w219) -> ("Numeric"=w220:dbl)  [unwired: 9 in, 1 out]
                n111 = call <vilib>:"NT Read String.vi"("Name"=w218) -> ("String"=w221:string)  [unwired: 9 in, 1 out]
                n112 = Bundle("Numeric"=w220, "String"=w221) -> (→"Progress":cluster{"Numeric":dbl, "String":string})  [unwired: 1 in]
              }
              frame "" {
                n113 = property on="Progress" class="Clust (strict)"("Visible"=FALSE) -> ()  [unwired: 2 in, 2 out]
                n114 = local write "Test Name"(u16 0) -> ()
              }
            }
            n115 = property on="Test Tree" class="Tree (strict)"("Active Item Row Number"=w215, "ActiveColNum"=w215, "CellBG"=w212, "Active Item Row Number"=-1 ("Active Item:Row Number"), "CellBG"=u32 5789784 ("Color Box")) -> ()  [unwired: 2 in, 2 out]
          }
          frame "Variables" {
            w227 = string[] ["CameraPublisher", "Usage", "DB"]  # Items to initially close
            n116 = First Call?() -> (First Call?: T/F=w228:bool)
            n117 = control-ref of="Tree"() -> (w229:refnum<vi>)
            n118 = Select(t=w227, s=w228, f=string[] []) -> (s? t:f=w225:string[])
            n119 = call <vilib>:"NT Read and Format Entries as Tree.vi"("Tags to  Close"=w225, "Tree Refnum"=w229) -> ()  [unwired: 8 in, 2 out]
          }
          frame "Commands" {
            w238 = u32 5789784 ("Color Box")
            w239 = T24 {"Row"=-1, "Column"=-2} ("Active Cell:Active Cell")
            w241 = T24 {"Row"=-2, "Column"=-2} ("Active Cell:Active Cell")
            n120 = Index Array(array=w242, index=w236) -> (element=w240:u32)
            n121 = Index Array(array=w237, index=w236) -> (element=w235:T23)
            n122 = Unbundle(w235) -> ("Operation"=w234:enum16{"Update", "Clear"})  [unwired: 1 out]
            n123 = local read "Command Selection"() -> (w233:i32)
            n124 = property on="Command Selection" class="MCListbox (strict)"("ActiveCell"=w241, "CellBG"=w240, "ActiveCell"=w239, "CellBG"=w238) -> ()  [unwired: 2 in, 2 out]
            n125 = call <vilib>:"WPI_DashboardUpdate RPC Info.vi"("Operation"=w234) -> ("update"=w232:bool, "commands"=w231:string[][])  [unwired: 9 in]
            n126 = property on="Command Selection" class="MCListbox (strict)"("ItemNames"=w231) -> ()  [unwired: 2 in, 2 out]
            n127 = property on="Command Params" class="Tbl (strict)"("Active Cell"=w241, "Cell BG Color"=w240, "Active Cell"=w239, "Cell BG Color"=w238) -> ()  [unwired: 2 in, 2 out]
            n128 = call <vilib>:"WPI_DashboardUpdate Command Params.vi"("Update"=w232, "NewVal"=w233, "Commands"=w231, "Param Tbl"=w230) -> ()  [unwired: 7 in, 1 out]
          }
        }
        n129 = call <vilib>:"Connextion Info.vi"() -> ("Connected"=→"NT Connection":bool)  [unwired: 10 in, 1 out]
      }
      event "Test Tree": Value Change {
        # "Show appropriate\ncontrols"
        n130 = event-data() -> ("CtlRef"=w247:refnum<vi>, "NewVal"=w245:string)  [unwired: 1 in]
        n131 = call <vilib>:"WPI_UtilitiesGetTreeIOName.vi"("NewVal"=w245, "TreeControl in"=w247) -> ("I/O Name"=w248:string)  [unwired: 9 in]
        n132 = case shown="\"Camera\"" w248 {
          selector: w248 -> [_ w255 _ w277 w286 _]
          tunnel: w245 -> [_ _ w274 w276 _ w293]
          tunnel: cluster{string[]}[] [{["640x480", "320x240", "160x120"]}, {["Auto", "Fixed indoor", "Fixed outdoor 1", "Fixed outdoor 2", "Fixed fluorescent 1", "Fixed fluorescent 2", "Hold current"]}, {["Auto", "Flicker-free 50 Hz", "Flicker-free 60 Hz", "Hold current"]}, {["None", "Prioritize frame rate", "Prioritize image quality"]}, {["Monochrome", "Color"]}] -> [_ _ _ _ _ w292]
          frame Default {
            w250 = FALSE ("Visible")
            w249 = FALSE ("Visible")
            n133 = property on="Motor" class="Clust (strict)"("Visible"=w249) -> ()  [unwired: 2 in, 2 out]
            n134 = property on="Test Ring" class="Ring (strict)"("Visible"=w249) -> ()  [unwired: 2 in, 2 out]
            n135 = property on="Rev/Fwd" class="Clust (strict)"("Visible"=w250) -> ()  [unwired: 2 in, 2 out]
            n136 = property on="On/Off" class="Bool (strict)"("Visible"=w250) -> ()  [unwired: 2 in, 2 out]
            n137 = property on="Test Slider" class="Slide (strict)"("Visible"=w250) -> ()  [unwired: 2 in, 2 out]
          }
          frame "Analog Out", "Motor", "PWM" {
            w256 = FALSE ("Visible")
            n138 = case shown="\"Analog Out\"" w255 {
              tunnel: [1.0 ("Value") -1.0 ("Value") 0.0 ("Value")] -> w254
              tunnel: [255.0 ("Value") 1.0 ("Value") 5.0 ("Value")] -> w253
              tunnel: [128.0 ("Value") 0.0 ("Value") 0.0 ("Value")] -> w252
              tunnel: [64.0 ("Value") 0.5 ("Value") 1.0 ("Value")] -> w251
              frame "PWM" {
              }
              frame "Motor", Default {
              }
              frame "Analog Out" {
              }
            }
            n139 = property on="Motor" class="Clust (strict)"("Visible"=TRUE) -> ()  [unwired: 2 in, 2 out]
            n140 = property on="Value" class="Slide (strict)"("Value"=w252, "Scale.Minimum"=w254, "Scale.Maximum"=w253, "Scale.Increment"=w251) -> ()  [unwired: 2 in, 2 out]
            n141 = property on="On/Off" class="Bool (strict)"("Visible"=w256) -> ()  [unwired: 2 in, 2 out]
            n142 = property on="Test Slider" class="Slide (strict)"("Visible"=w256) -> ()  [unwired: 2 in, 2 out]
            n143 = property on="Test Ring" class="Ring (strict)"("Visible"=w256) -> ()  [unwired: 2 in, 2 out]
            n144 = property on="Rev/Fwd" class="Clust (strict)"("Visible"=w256) -> ()  [unwired: 2 in, 2 out]
          }
          frame "Servo" {
            w272 = FALSE ("Visible")
            n145 = call <vilib>:"NT Read Number.vi"("Name"=w274) -> ("Numeric"=w273:dbl)  [unwired: 9 in, 1 out]
            n146 = property on="Test Slider" class="Slide (strict)"("Visible"=TRUE, "Scale.Maximum"=170.0 ("Scale.Range:Maximum")) -> ()  [unwired: 2 in, 2 out]
            n147 = local write "Test Slider"(w273) -> ()
            n148 = property on="Motor" class="Clust (strict)"("Visible"=w272) -> ()  [unwired: 2 in, 2 out]
            n149 = property on="Rev/Fwd" class="Clust (strict)"("Visible"=w272) -> ()  [unwired: 2 in, 2 out]
            n150 = property on="On/Off" class="Bool (strict)"("Visible"=w272) -> ()  [unwired: 2 in, 2 out]
            n151 = property on="Test Ring" class="Ring (strict)"("Visible"=w272) -> ()  [unwired: 2 in, 2 out]
          }
          frame "Relay", "Solenoid" {
            w275 = FALSE ("Visible")
            n152 = property on="Motor" class="Clust (strict)"("Visible"=w275) -> ()  [unwired: 2 in, 2 out]
            n153 = property on="Test Slider" class="Slide (strict)"("Visible"=w275) -> ()  [unwired: 2 in, 2 out]
            n154 = Search and Replace String(input string=w276, search string="/Value  **", replace string="/Direction") -> (result string=w282:string)  [unwired: 5 in, 3 out]
            n155 = property on="Test Ring" class="Ring (strict)"("Visible"=w275) -> ()  [unwired: 2 in, 2 out]
            n156 = call <vilib>:"NT Read String.vi"("Name"=w282) -> ("String"=w280:string)  [unwired: 9 in, 1 out]
            n157 = Equal?(x="Both directions", y=w280) -> (x = y?=w278:bool)
            n158 = Not(x=w278) -> (.not. x?=w279:bool)
            n159 = property on="Rev/Fwd" class="Clust (strict)"("Visible"=w278) -> ()  [unwired: 2 in, 2 out]
            n160 = property on="On/Off" class="Bool (strict)"("Visible"=w279, "Caption.Text"=w277) -> ()  [unwired: 2 in, 2 out]
          }
          frame "Compressor", "Digital Out" {
            w285 = FALSE ("Visible")
            # "Get direction and finish"
            n161 = property on="Motor" class="Clust (strict)"("Visible"=w285) -> ()  [unwired: 2 in, 2 out]
            n162 = property on="Test Slider" class="Slide (strict)"("Visible"=w285) -> ()  [unwired: 2 in, 2 out]
            n163 = property on="Test Ring" class="Ring (strict)"("Visible"=w285) -> ()  [unwired: 2 in, 2 out]
            n164 = property on="On/Off" class="Bool (strict)"("Visible"=TRUE, "Caption.Text"=w286) -> ()  [unwired: 2 in, 2 out]
            n165 = property on="Rev/Fwd" class="Clust (strict)"("Visible"=FALSE) -> ()  [unwired: 2 in, 2 out]
          }
          frame "Camera" {
            n166 = call <vilib>:"Get Last Path Segment.vi"("String in"=w293) -> ("String out"=w294:string)  [unwired: 10 in]
            n167 = property on="On/Off" class="Bool (strict)"("Visible"=FALSE) -> ()  [unwired: 2 in, 2 out]
            n168 = property on="Motor" class="Clust (strict)"("Visible"=FALSE) -> ()  [unwired: 2 in, 2 out]
            n169 = property on="Rev/Fwd" class="Clust (strict)"("Visible"=FALSE) -> ()  [unwired: 2 in, 2 out]
            n170 = case shown="\"White Balance  **\"" w294 {
              tunnel: w293 -> [w300 w309 w318 w327 w336 _ w342]
              tunnel: w292 -> [w298 w306 w315 w324 w333 _ _]
              frame "Size  **" {
                n171 = Index Array(array=w298) -> (element=w297:cluster{string[]})  [unwired: 1 in]
                n172 = call <vilib>:"NT Read String.vi"("Name"=w300) -> ("String"=w299:string)  [unwired: 9 in, 1 out]
                n173 = Unbundle(w297) -> (w295:string[])
                n174 = Match First String(2:w295, 3:w299) -> (0:w296:i32)  [unwired: 1 out]
                n175 = property on="Test Ring" class="Ring (strict)"("Value"=w296, "Strings []"=w295) -> ()  [unwired: 2 in, 2 out]
                n176 = property on="Test Ring" class="Ring (strict)"("Visible"=TRUE) -> ()  [unwired: 2 in, 2 out]
                n177 = property on="Test Slider" class="Slide (strict)"("Visible"=FALSE) -> ()  [unwired: 2 in, 2 out]
              }
              frame "White Balance  **" {
                n178 = Index Array(array=w306, index=1) -> (element=w307:cluster{string[]})
                n179 = call <vilib>:"NT Read String.vi"("Name"=w309) -> ("String"=w308:string)  [unwired: 9 in, 1 out]
                n180 = Unbundle(w307) -> (w304:string[])
                n181 = Match First String(2:w304, 3:w308) -> (0:w303:i32)  [unwired: 1 out]
                n182 = property on="Test Ring" class="Ring (strict)"("Value"=w303, "Strings []"=w304) -> ()  [unwired: 2 in, 2 out]
                n183 = property on="Test Ring" class="Ring (strict)"("Visible"=TRUE) -> ()  [unwired: 2 in, 2 out]
                n184 = property on="Test Slider" class="Slide (strict)"("Visible"=FALSE) -> ()  [unwired: 2 in, 2 out]
              }
              frame "Exposure  **" {
                n185 = Index Array(array=w315, index=2) -> (element=w316:cluster{string[]})
                n186 = call <vilib>:"NT Read String.vi"("Name"=w318) -> ("String"=w317:string)  [unwired: 9 in, 1 out]
                n187 = Unbundle(w316) -> (w312:string[])
                n188 = Match First String(2:w312, 3:w317) -> (0:w313:i32)  [unwired: 1 out]
                n189 = property on="Test Ring" class="Ring (strict)"("Value"=w313, "Strings []"=w312) -> ()  [unwired: 2 in, 2 out]
                n190 = property on="Test Ring" class="Ring (strict)"("Visible"=TRUE) -> ()  [unwired: 2 in, 2 out]
                n191 = property on="Test Slider" class="Slide (strict)"("Visible"=FALSE) -> ()  [unwired: 2 in, 2 out]
              }
              frame "Exposure Priority  **" {
                n192 = Index Array(array=w324, index=3) -> (element=w325:cluster{string[]})
                n193 = call <vilib>:"NT Read String.vi"("Name"=w327) -> ("String"=w326:string)  [unwired: 9 in, 1 out]
                n194 = Unbundle(w325) -> (w321:string[])
                n195 = Match First String(2:w321, 3:w326) -> (0:w322:i32)  [unwired: 1 out]
                n196 = property on="Test Ring" class="Ring (strict)"("Value"=w322, "Strings []"=w321) -> ()  [unwired: 2 in, 2 out]
                n197 = property on="Test Ring" class="Ring (strict)"("Visible"=TRUE) -> ()  [unwired: 2 in, 2 out]
                n198 = property on="Test Slider" class="Slide (strict)"("Visible"=FALSE) -> ()  [unwired: 2 in, 2 out]
              }
              frame "Color Enable  **" {
                n199 = Index Array(array=w333, index=4) -> (element=w334:cluster{string[]})
                n200 = call <vilib>:"NT Read String.vi"("Name"=w336) -> ("String"=w335:string)  [unwired: 9 in, 1 out]
                n201 = Unbundle(w334) -> (w330:string[])
                n202 = Match First String(2:w330, 3:w335) -> (0:w331:i32)  [unwired: 1 out]
                n203 = property on="Test Ring" class="Ring (strict)"("Value"=w331, "Strings []"=w330) -> ()  [unwired: 2 in, 2 out]
                n204 = property on="Test Ring" class="Ring (strict)"("Visible"=TRUE) -> ()  [unwired: 2 in, 2 out]
                n205 = property on="Test Slider" class="Slide (strict)"("Visible"=FALSE) -> ()  [unwired: 2 in, 2 out]
              }
              frame Default {
                n206 = property on="Test Ring" class="Ring (strict)"("Visible"=FALSE) -> ()  [unwired: 2 in, 2 out]
                n207 = property on="Test Slider" class="Slide (strict)"("Visible"=FALSE) -> ()  [unwired: 2 in, 2 out]
              }
              frame "Brightness  **", "Color Level  **", "Compression  **", "FPS  **", "Sharpness  **" {
                n208 = call <vilib>:"NT Read Number.vi"("Name"=w342) -> ("Numeric"=w341:dbl)  [unwired: 9 in, 1 out]
                n209 = local write "Test Slider"(w341) -> ()
                n210 = property on="Test Ring" class="Ring (strict)"("Visible"=FALSE) -> ()  [unwired: 2 in, 2 out]
                n211 = property on="Test Slider" class="Slide (strict)"("Visible"=TRUE, "Scale.Maximum"=100.0 ("Scale.Range:Maximum")) -> ()  [unwired: 2 in, 2 out]
              }
            }
          }
        }
        n212 = property on="Progress" class="Clust (strict)"("Visible"=FALSE) -> ()  [unwired: 2 in, 2 out]
      }
      event "Test Name": Mouse Enter {
        # "Populate the ring with the list of tests"
        n213 = event-data() -> ()  [unwired: 1 in, 1 out]
        n214 = call <vilib>:"NT Read String Array.vi"("Name"="TestMode/TestList") -> ("String Array"=w350:string[])  [unwired: 9 in, 1 out]
        n215 = Build Array (concatenate)("Select the test to run...", w350) -> (w349:string[])
        n216 = property on="Test Name" class="Ring (strict)"("Strings []"=w349) -> ()  [unwired: 2 in, 2 out]
      }
      event "Test Name": Value Change {
        w352 = FALSE ("Visible")
        # "Tell the robot the test name to run"
        n217 = event-data() -> ("NewVal"=w356:u16)  [unwired: 1 in]
        n218 = property on="Test Name" class="Ring (strict)"() -> ("Strings []"=w357:string[])  [unwired: 2 in, 2 out]
        n219 = local write "Progress"(T6 {"Test Progress"=0, "Test Progress Text"=""} ("Progress")) -> ()
        n220 = Index Array(array=w357, index=w356) -> (element=w355:string)
        n221 = call <vilib>:"NT Write String.vi"("String"=w355, "Name"="TestMode/TestName") -> ()  [unwired: 9 in, 1 out]
        n222 = property on="Progress" class="Clust (strict)"("Visible"=TRUE) -> ()  [unwired: 2 in, 2 out]
        n223 = property on="Motor" class="Clust (strict)"("Visible"=w352) -> ()  [unwired: 2 in, 2 out]
        n224 = property on="Test Slider" class="Slide (strict)"("Visible"=w352) -> ()  [unwired: 2 in, 2 out]
        n225 = property on="On/Off" class="Bool (strict)"("Visible"=w352) -> ()  [unwired: 2 in, 2 out]
        n226 = property on="Rev/Fwd" class="Clust (strict)"("Visible"=w352) -> ()  [unwired: 2 in, 2 out]
        n227 = property on="Test Ring" class="Ring (strict)"("Visible"=w352) -> ()  [unwired: 2 in, 2 out]
      }
      event "Select Auto": Mouse Enter {
        # "Populate the combo box with the list of autonomous options"
        n228 = event-data() -> ()  [unwired: 1 in, 1 out]
        n229 = call <vilib>:"NT Read String Array.vi"("Name"="Auto List") -> ("String Array"=w359:string[])  [unwired: 9 in, 1 out]
        n230 = property on="Select Auto" class="CmbBox"("Strings[]"=w359) -> ()  [unwired: 2 in, 2 out]
      }
      event "Select Auto": Value Change {
        # "User modified the Auto Selection. Write to NT variable so robot knows."
        n231 = event-data() -> ("NewVal"=w362:string)  [unwired: 1 in]
        n232 = call <vilib>:"NT Write String.vi"("String"=w362, "Name"="Auto Selector") -> ()  [unwired: 9 in, 1 out]
      }
      event "Command Selection": Value Change {
        # "Get the params and show in table"
        n233 = event-data() -> ("NewVal"=w368:i32)  [unwired: 1 in]
        n234 = property on="Command Selection" class="MCListbox (strict)"() -> ("ItemNames"=w366:string[][])  [unwired: 2 in, 2 out]
        n235 = call <vilib>:"WPI_DashboardUpdate Command Params.vi"("NewVal"=w368, "Commands"=w366, "Param Tbl"=w367) -> ()  [unwired: 8 in, 1 out]
      }
      event "Execute Command": Value Change {
        # "Started one, Unique ID holds\nresponse"
        n236 = event-data() -> ()  [unwired: 1 in, 1 out]
        n237 = property on="Command Selection" class="MCListbox (strict)"() -> ("ItemNames"=w379:string[][])  [unwired: 2 in, 2 out]
        n238 = Index Array(array=w379, index (row)="Command Selection", index (col)=0) -> (element=w377:string)
        n239 = call <vilib>:"Invoke Commands.vi"("Command Params"="Command Params", "Function Name"=w377) -> ("Params"=w373:u8, "Started"=w372:bool)  [unwired: 7 in, 1 out]
        n240 = Array Subset(array="Command Params", length (row)=w373) -> (w374:string[][])  [unwired: 3 in]
        n241 = Select(t="Executing" ("Cmd Status"), s=w372, f="" ("Cmd Status")) -> (s? t:f=→"Cmd Status":string)
      }
      event "Command Selection": Double Click {
        n242 = event-data() -> ("Row"=w387:i32)  [unwired: 1 in]
        n243 = property on="Command Selection" class="MCListbox (strict)"() -> ("ItemNames"=w390:string[][])  [unwired: 2 in, 2 out]
        n244 = local read "Command Params"() -> (w386:string[][])
        n245 = Index Array(array=w390, index (row)=w387, index (col)=0) -> (element=w388:string)
        n246 = call <vilib>:"Invoke Commands.vi"("Command Params"=w386, "Function Name"=w388) -> ("Params"=w385:u8, "Started"=w380:bool)  [unwired: 7 in, 1 out]
        n247 = Array Subset(array=w386, length (row)=w385) -> (w384:string[][])  [unwired: 3 in]
        n248 = Select(t="Executing" ("Cmd Status"), s=w380, f="" ("Cmd Status")) -> (s? t:f=w381:string)
        n249 = local write "Cmd Status"(w381) -> ()
      }
      event "CheckList": Double Click {
        # "Shift clears all"
        # "Update symbols on the listbox"
        n250 = event-data() -> ("PlatMods.Shift"=w392:bool, "Row"=w394:i32)  [unwired: 1 in]
        n251 = case shown="True" w392 {
          tunnel: w394 -> [w398 _]
          tunnel: 1 -> [w397 _]
          frame False {
            n252 = property on="CheckList" class="LstBox (strict)"() -> ("Item Symbols"=w396:i32[])  [unwired: 2 in, 2 out]
            n253 = Replace Array Subset(array=w396, new element=w397, index=w398) -> (w395:i32[])
            n254 = property on="CheckList" class="LstBox (strict)"("Item Symbols"=w395) -> ()  [unwired: 2 in, 2 out]
          }
          frame True {
            w399 = 0 ("Top Row")
            n255 = property on="CheckList" class="LstBox (strict)"() -> ("Number of Rows"=w401:u32)  [unwired: 2 in, 2 out]
            n256 = Initialize Array(0, w401) -> (w400:i32[])
            n257 = property on="CheckList" class="LstBox (strict)"("Top Row"=w399, "Value"=w399, "Item Symbols"=w400) -> ()  [unwired: 2 in, 2 out]
          }
        }
      }
      event "CheckList": Key Down {
        # "Update symbols on the listbox\nLeft and right keys check and uncheck"
        n258 = event-data() -> ("VKey"=w405:T21)  [unwired: 1 in]
        n259 = case shown="\"Left\", \"Right\"" w405 {
          selector: w405 -> [w410 _]
          tunnel: eventvkey."Left" ("VKey") -> [w408 _]
          frame "Left", "Right" {
            n260 = Equal?(x=w408, y=w410) -> (x = y?=w409:bool)
            n261 = Select(t=0, s=w409, f=1) -> (s? t:f=w411:i32)
            n262 = property on="CheckList" class="LstBox (strict)"() -> ("Item Symbols"=w414:i32[])  [unwired: 2 in, 2 out]
            n263 = Replace Array Subset(array=w414, new element=w411, index="CheckList") -> (w413:i32[])
            n264 = property on="CheckList" class="LstBox (strict)"("Item Symbols"=w413) -> ()  [unwired: 2 in, 2 out]
          }
          frame Default {
          }
        }
      }
      event "Motor.Enable": Value Change {
        # "When the test mode otor enable helper is set, update that\ntree row item's value"
        n265 = event-data() -> ("NewVal"=w420:bool)  [unwired: 1 in]
        n266 = Unbundle("Motor") -> ("Value"=w419:dbl)  [unwired: 1 out]
        n267 = Select(t=w419, s=w420, f=0.0) -> (s? t:f=w417:dbl)
        n268 = call <vilib>:"NT Write Number.vi"("Numeric"=w417, "Name"=w416) -> ()  [unwired: 9 in, 1 out]
      }
      event "Test Slider": Value Change {
        # "When the test mode slider helper is set, update that\ntree row item's value"
        n269 = event-data() -> ("NewVal"=w423:dbl)  [unwired: 1 in]
        n270 = call <vilib>:"NT Write Number.vi"("Numeric"=w423, "Name"=w424) -> ()  [unwired: 9 in, 1 out]
      }
      event "On/Off": Value Change {
        # "When the test mode on/off helper value is set, update that\ntree row item's value"
        n271 = event-data() -> ("NewVal"=w428:bool)  [unwired: 1 in]
        n272 = Boolean To (0,1)(Boolean=w428) -> (0, 1=w427:i16)
        n273 = call <vilib>:"NT Write Number.vi"("Numeric"=w427, "Name"=w426) -> ()  [unwired: 9 in, 1 out]
      }
      event "Rev/Fwd": Value Change {
        # "When the test mode helper value for relays is set, update that\ntree row item's value"
        n274 = event-data() -> ("NewVal.Forward"=w436:bool, "NewVal.Reverse"=w435:bool)  [unwired: 1 in]
        n275 = Boolean To (0,1)(Boolean=w436) -> (0, 1=w432:i16)
        n276 = Boolean To (0,1)(Boolean=w435) -> (0, 1=w434:i16)
        n277 = Negate(x=w434) -> (-x=w433:i16)
        n278 = Add(x=w432, y=w433) -> (x+y=w431:i16)
        n279 = call <vilib>:"NT Write Number.vi"("Numeric"=w431, "Name"=w430) -> ()  [unwired: 9 in, 1 out]
      }
      event "Test Ring": Value Change {
        # "When a test mode helper value is selected from the ring,\nset the tree item's variable to the string value"
        n280 = event-data() -> ("NewVal"=w440:u16)  [unwired: 1 in]
        n281 = property on="Test Ring" class="Ring (strict)"() -> ("Strings []"=w441:string[])  [unwired: 2 in, 2 out]
        n282 = Index Array(array=w441, index=w440) -> (element=w439:string)
        n283 = call <vilib>:"NT Write String.vi"("String"=w439, "Name"=w438) -> ()  [unwired: 9 in, 1 out]
      }
      event "Rec Mode": Value Change {
        # "Update globals for recording mode and path to read log from.\nClear when logging and let NetworkTables set path for vision to\nuse."
        n284 = event-data() -> ("NewVal"=w452:enum32{"Stop", "Record", "Playback"})  [unwired: 1 in]
        n285 = global write "WPI_DashboardLogging Global.vi" "Recording"(w452) -> ()
        n286 = global write "WPI_DashboardLogging Global.vi" "Logging Filename"(path "") -> ()
        n287 = case shown="\"Playback\"" w452 {
          tunnel: w451 -> [_ w454 w463]
          tunnel: [_ _ w462] -> w449
          tunnel: [_ _ w461] -> _
          tunnel: w447 -> [_ _ w459]
          tunnel: cluster{i32, i32} {-250, 170} -> [_ _ w458]
          tunnel: [_ _ T22 {"Image Size"=TRUE, "Image Type"=TRUE, "Pixel Value"=TRUE, "ROI Information"=TRUE, "Zoom Factor"=FALSE} ("Image Information Shown:All Elements")] -> w442
          tunnel: [_ _ TRUE ("Zoom Factor")] -> w443
          tunnel: w445 -> [_ _ w455]
          frame Default {
          }
          frame "Stop", "Record" {
            # "Place Window too"
            n288 = invoke class="VI" method="FP.Close"(reference=w454) -> (reference out=w453:refnum<vi>)  [unwired: 2 in, 2 out]
            n289 = invoke class="VI" method="Abort VI"(reference=w453) -> ()  [unwired: 2 in, 3 out]
          }
          frame "Playback" {
            n290 = call "Open Playback Panel.vi"("Offset"=w458, "DB VI Ref"=w459, "Playback in"=w463) -> ("Playback out"=w460:refnum<vi>)  [unwired: 8 in]
            n291 = register-events(w460, w455) -> (reference out=w462:refnum<event-registration>, error out=w461:errorcluster)  [unwired: 2 in]
          }
        }
        n292 = property on="Camera Image Right" class="ImageControl"("Image Information Shown"=w442, "Image Information Visible"=w443) -> ()  [unwired: 2 in, 2 out]
        n293 = property on="Camera Image" class="ImageControl"("Image Information Shown"=w442, "Image Information Visible"=w443) -> ()  [unwired: 2 in, 2 out]
        n294 = call <vilib>:"WPI_DashboardNT Log FieldName Cache.vi"("Operation"=enum16{"Lookup/Add", "Index", "Clear"}."Clear") -> ()  [unwired: 8 in, 3 out]
      }
      event Panel Close {
        w465 = enum32{"Stop", "Record", "Playback"}."Stop" ("Rec Mode")
        # "Playback window has been closed, abort"
        n295 = event-data() -> ()  [unwired: 1 in, 4 out]
        n296 = local write "Rec Mode"(w465) -> ()
        n297 = global write "WPI_DashboardLogging Global.vi" "Recording"(w465) -> ()
      }
      event Panel Close {
        # "Abort playback window and ourself"
        n298 = event-data() -> ()  [unwired: 1 in, 4 out]
        n299 = invoke class="VI" method="FP.Close"(reference=w469) -> (reference out=w468:refnum<vi>)  [unwired: 2 in, 2 out]
        n300 = invoke class="VI" method="Abort VI"(reference=w468) -> (error out=w467:errorcluster)  [unwired: 2 in, 2 out]
        n301 = invoke class="VI" method="Abort VI"(error in=w467) -> ()  [unwired: 2 in, 3 out]
      }
      event User Event {
        n302 = event-data() -> ("IDs"=w476:cluster{"RPC field ID":u16, "Unique ID":u16}, "String"=w475:string)  [unwired: 1 in]
        n303 = Bundle("IDs"=w476, "String"=w475) -> (w474:T9)  [unwired: 1 in]
        n304 = call <vilib>:"Retrieve RPC Response.vi"("RPC Response"=w474) -> ("Output"=w472:string[][])  [unwired: 10 in]
        n305 = Build Array (concatenate)(w470, w472) -> (w471:string[][])
        n306 = local write "Command Params"(w471) -> ()
        n307 = local write "Cmd Status"("" ("Cmd Status")) -> ()
      }
      event "Tree": Double Click {
        n308 = event-data() -> ("PlatMods"=w482:T25, "Tag"=w479:string)  [unwired: 1 in]
        n309 = Unbundle(w482) -> ("Shift"=w481:bool)  [unwired: 4 out]
        n310 = String Subset(string=w479, length (rest)=1 ("length (rest)")) -> (substring=w478:string)  [unwired: 1 in]
        n311 = Not(x=w481) -> (.not. x?=w480:bool)
        n312 = case shown="\"/\"" w478 {
          tunnel: w479 -> [_ w485]
          tunnel: w480 -> [_ w484]
          frame Default {
          }
          frame "/" {
            n313 = call <vilib>:"NT Update Persistence.vi"("Persistence"=w484, "Name"=w485) -> ()  [unwired: 9 in, 1 out]
          }
        }
      }
    }
  }
  n314 = while {
    tunnel: w65 -> [w487]
    i -> [w490]
    stop <- FALSE stop-if-true
    n315 = Wait (ms)(milliseconds to wait=u32 100) -> ()  [unwired: 1 out]
    n316 = case shown="\"Playback\"" "Rec Mode" {
      tunnel: w490 -> [_ _ w505]
      tunnel: [u32 2829099 ("Base Color") u32 11141120 ("Target Color") w494] -> w486
      frame "Stop", Default {
        # "Reset the color, extra updates don't cost much"
      }
      frame "Record" {
      }
      frame "Playback" {
        # "Playback"
        n317 = Quotient & Remainder(x=w505, y=u32 50 ("milliseconds to wait")) -> (x-y*floor(x/y)=w501:u32)  [unwired: 1 out]
        n318 = Divide(x=w501, y=u32 50 ("milliseconds to wait")) -> (x/y=w498:dbl)
        n319 = Multiply(x=6.283185307179586, y=w498) -> (x*y=w503:dbl)
        n320 = Sine(x=w503) -> (sin(x)=w502:dbl)
        n321 = Absolute Value(x=w502) -> (abs(x)=w495:dbl)
        n322 = call "Interpolate RGB Color.vi"("Proportion"=w495, "Target Color"=u32 30976, "Base Color"=u32 2829099) -> ("Result Color"=w494:u32)  [unwired: 8 in]
      }
    }
    n323 = property class="Pane"(reference=w487, "PaneColor"=w486) -> ()  [unwired: 1 in, 2 out]
  }
  n324 = local write "Dashboard Tab"(T2."Drive" ("Dashboard Tab")) -> ()
  n325 = property on="On/Off" class="Bool (strict)"("Visible"=w36) -> ()  [unwired: 2 in, 2 out]
  n326 = property on="Motor" class="Clust (strict)"("Visible"=w36) -> ()  [unwired: 2 in, 2 out]
  n327 = property on="Progress" class="Clust (strict)"("Visible"=w36) -> ()  [unwired: 2 in, 2 out]
  n328 = property on="Test Ring" class="Ring (strict)"("Visible"=w36) -> ()  [unwired: 2 in, 2 out]
  n329 = property on="Rev/Fwd" class="Clust (strict)"("Visible"=w36) -> ()  [unwired: 2 in, 2 out]
  n330 = while {
    tunnel: u16 1741 ("timeout ms (25000)") -> [w507]
    stop <- FALSE stop-if-true
    n331 = TCP Create Listener(10:w507) -> (0:w506:errorcluster, 3:w508:refnum<k5>)  [unwired: 4 in, 1 out]
    n332 = case shown="No Error" w506 {
      selector: w506 -> [w510 _]
      tunnel: w508 -> [w511 _]
      frame No Error {
        n333 = while {
          tunnel: w511 -> [w514]
          tunnel: w510 -> [w513]
          stop <- FALSE stop-if-true
          n334 = TCP Wait On Listener(8:w513, 11:w514) -> (0:w515:errorcluster, 4:w516:refnum<k5>)  [unwired: 2 in, 3 out]
          n335 = local write "TCP"(w516) -> ()
          n336 = case shown="No Error" w515 {
            frame No Error {
            }
            frame Error {
              n337 = Wait (ms)(milliseconds to wait=u32 1000) -> ()  [unwired: 1 out]
            }
          }
        }
      }
      frame Error {
        n338 = Wait (ms)(milliseconds to wait=u32 1000) -> ()  [unwired: 1 out]
      }
    }
  }
  n339 = local write "Command Selection"(u16 0 ("milliseconds to wait")) -> ()
  n340 = local write "Command Params"(string[][] [] ("Command Params")) -> ()
  n341 = global write "WPI_DashboardLogging Global.vi" "Recording"(w59) -> ()
  n342 = local write "Rec Mode"(w59) -> ()
  n343 = call <vilib>:"NT Write String.vi"("String"="Select Auto", "Name"="Auto Selector") -> ()  [unwired: 9 in, 1 out]
